vi "NoDashDefaultToValue.vi"(1 "Numeric 2":dbl, 2 "Numeric":dbl) -> (0 "Numeric 3":dbl)   [LabVIEW 2013]
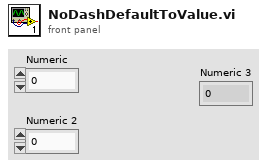
[diagram p1: front panel]
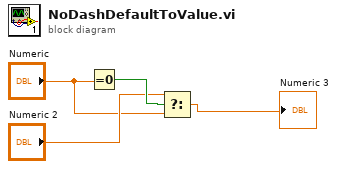
[diagram p0: block diagram]
diagram:
  n1 = Equal To 0?(x="Numeric") -> (x = 0?=w4:bool)
  n2 = Select(t="Numeric 2", s=w4, f="Numeric") -> (s? t:f=→"Numeric 3":dbl)
